vi "SoundBeep.vi"(1 "Type":enum16{"Error", "Triple"}(ring)) -> ()   [LabVIEW 2014]
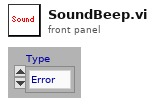
[diagram p1: front panel]
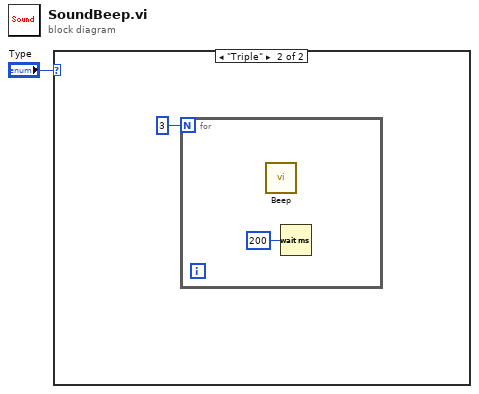
[diagram p0: block diagram]
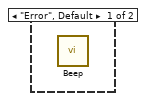
[diagram p2: hidden frame]
diagram:
  n1 = case shown="\"Triple\"" "Type" {
    frame "Error", Default {
      n2 = call <vilib>:"Beep.vi"() -> ()  [unwired: 12 in]
    }
    frame "Triple" {
      n3 = for {
        N: 3 -> [_]
        n4 = call <vilib>:"Beep.vi"() -> ()  [unwired: 12 in]
        n5 = Wait (ms)(milliseconds to wait=u32 200) -> ()  [unwired: 1 out]
      }
    }
  }
